vi "Host_GUI.vi"() -> ()   [LabVIEW 2017]
uses:
  <vilib>/Utility/miscctls.llb/LV3DPointTypeDef.ctl
  <vilib>/Analysis/coordinate.llb/Euler Rotation Order.ctl
  <vilib>/picture/3D Picture Control/Object/Create Object (drawable).vi
  <vilib>/picture/3D Picture Control/Object/Create Object (name).vi
  <vilib>/picture/3D Picture Control/Object/Add Object (no reference).vi
  <vilib>/picture/3D Picture Control/Helpers/Apply Texture (no reference).vi
  <vilib>/Analysis/NI_AALPro.lvlib
  <vilib>/picture/3D Picture Control/NI_3D Picture Control.lvlib
  <vilib>/picture/3D Picture Control/Helpers/Set Clip Plane (no reference).vi
panel:
  in  "Up Direction":T1={"X"=0.0, "Y"=0.0, "Z"=1.0}
  out "appended path":path
  in  "error in (no error)":errorcluster
  in  "N-frame rot":dbl[](array[numeric])
  in  "B-frame Translation 2":cluster{"X":sgl, "Y":sgl, "Z":sgl}
  out "B-frame [m]":cluster{"X":sgl, "Y":sgl, "Z":sgl}
  out "Enum":T2(ring)
  in  "Tab Control":enum32{"Inicialização", "Simulação"}(tab)
  in  "Simulation Parameters":T3={"Wind VelocityAzimuth [deg] "=0.0, "Wind Velocity Module [m/s]"=0.0, "Fe gain"=1.0, "Cnalpha gain"=1.0, "clp gain"=1.0, "cld gain"=1.0, "cmq gain"=1.0, "cnr gain"=1.0, "dl [º]"=0.0, "Nozzle misalignment yaw/pitch [º]"=[0.0, 0.0], "Nozzle eccentricity x/y [m]"=[], "Wind_Profile"=0} {"Wind_Profile" min=0 max=3 step=1; "Wind Velocity Module [m/s]" format="%#_13g"; "Wind VelocityAzimuth [deg]" format="%#_13g"}
  in  "Continuar":bool
  in  "stop":bool
  in  "Initialization Parameters":T4={"W_b ini [rad/s]"=[], "W ini [rad/s]"=[], "altitude_ini(m)"=50.0, "lon_ini [º]"=-44.3678, "latd_ini [º]"=-2.31599, "V_ini [m/s]"=[], "Initial Euler Angles [deg]"=[], "CFN-61G Enable"=FALSE, "Table enable"=FALSE, "DMARS Enable"=FALSE, "TVA Enable"=FALSE, "Sim_Time [s]"=82.0, "Control Selection"=enum."Sim Control"}
  out "Euler Angles [deg]":T5(graph)
  in  "Run_SIM":bool
  out "Sim_Stopped":bool
  in  "stop RT":bool
  out "Simulation time [s]":dbl
  out "Atitude":refnum<vi>(3d-picture)
  in  "stop GUI":bool
  out "floor(x/y)":dbl
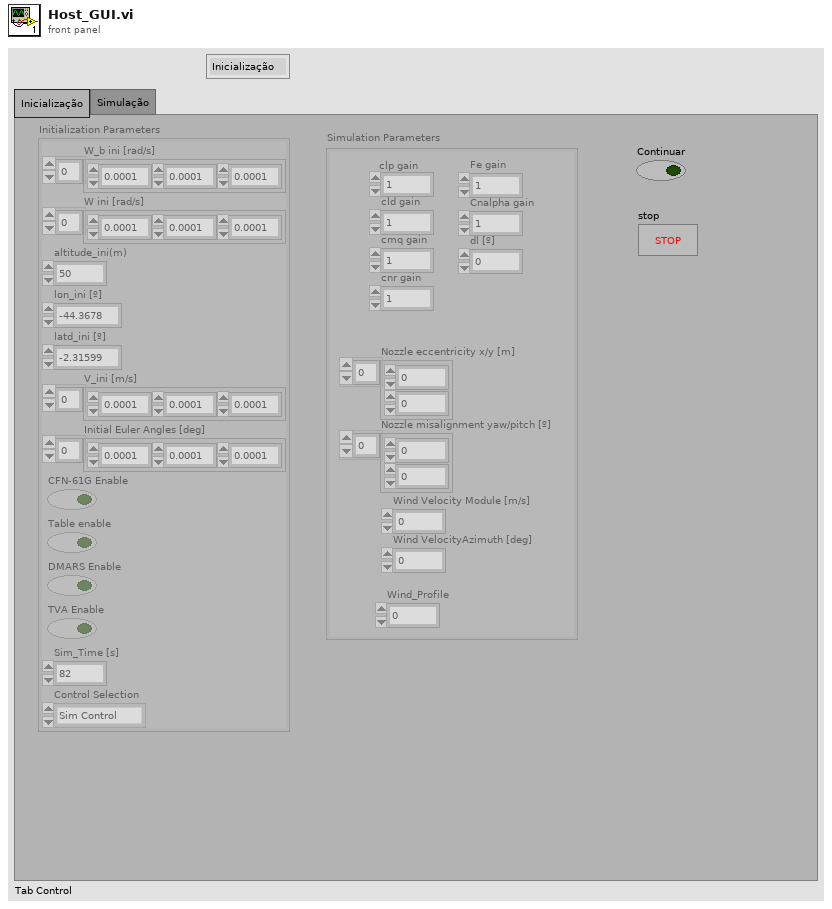
[diagram p1: front panel]
types:
  T1 = typedef "LV3DPointTypeDef.ctl" = cluster{"X":sgl, "Y":sgl, "Z":sgl}
  T2 = enum16{"Inicialização", "Simulação", "Resultados", "Finalizar RT"}
  T3 = cluster{"Wind VelocityAzimuth [deg] ":dbl, "Wind Velocity Module [m/s]":dbl, "Fe gain":dbl, "Cnalpha gain":dbl, "clp gain":dbl, "cld gain":dbl, "cmq gain":dbl, "cnr gain":dbl, "dl [º]":dbl, "Nozzle misalignment yaw/pitch [º]":dbl[], "Nozzle eccentricity x/y [m]":dbl[], "Wind_Profile":i32}
  T4 = cluster{"W_b ini [rad/s]":dbl[], "W ini [rad/s]":dbl[], "altitude_ini(m)":dbl, "lon_ini [º]":dbl, "latd_ini [º]":dbl, "V_ini [m/s]":dbl[], "Initial Euler Angles [deg]":dbl[], "CFN-61G Enable":bool, "Table enable":bool, "DMARS Enable":bool, "TVA Enable":bool, "Sim_Time [s]":dbl, "Control Selection":enum16{"Constant", "TVA E-BOX", "Sim Control"}}
  T5 = cluster{"Numeric":dbl, "Numeric":dbl, "Numeric":dbl}
  T6 = enum16{"As a Decal", "With Modulation", "With Blending", "As a replacement"}
  T7 = cluster{"Red":sgl, "Green":sgl, "Blue":sgl, "Alpha":sgl}
  T8 = enum8{"Enabled", "Disabled", "Disabled and Grayed Out"}
  T9 = typedef "NI_AALPro.lvlib/Euler Rotation Order.ctl" = u16
  T10 = typedef "imagedata.ctl" = cluster{"image type":i32, "image depth":i32, "image":u8[], "mask":u8[], "colors":u32[], "Rectangle":cluster{"left":i16, "top":i16, "right":i16, "bottom":i16}}
  T11 = cluster{"element":dbl, "element":dbl, "element":dbl}
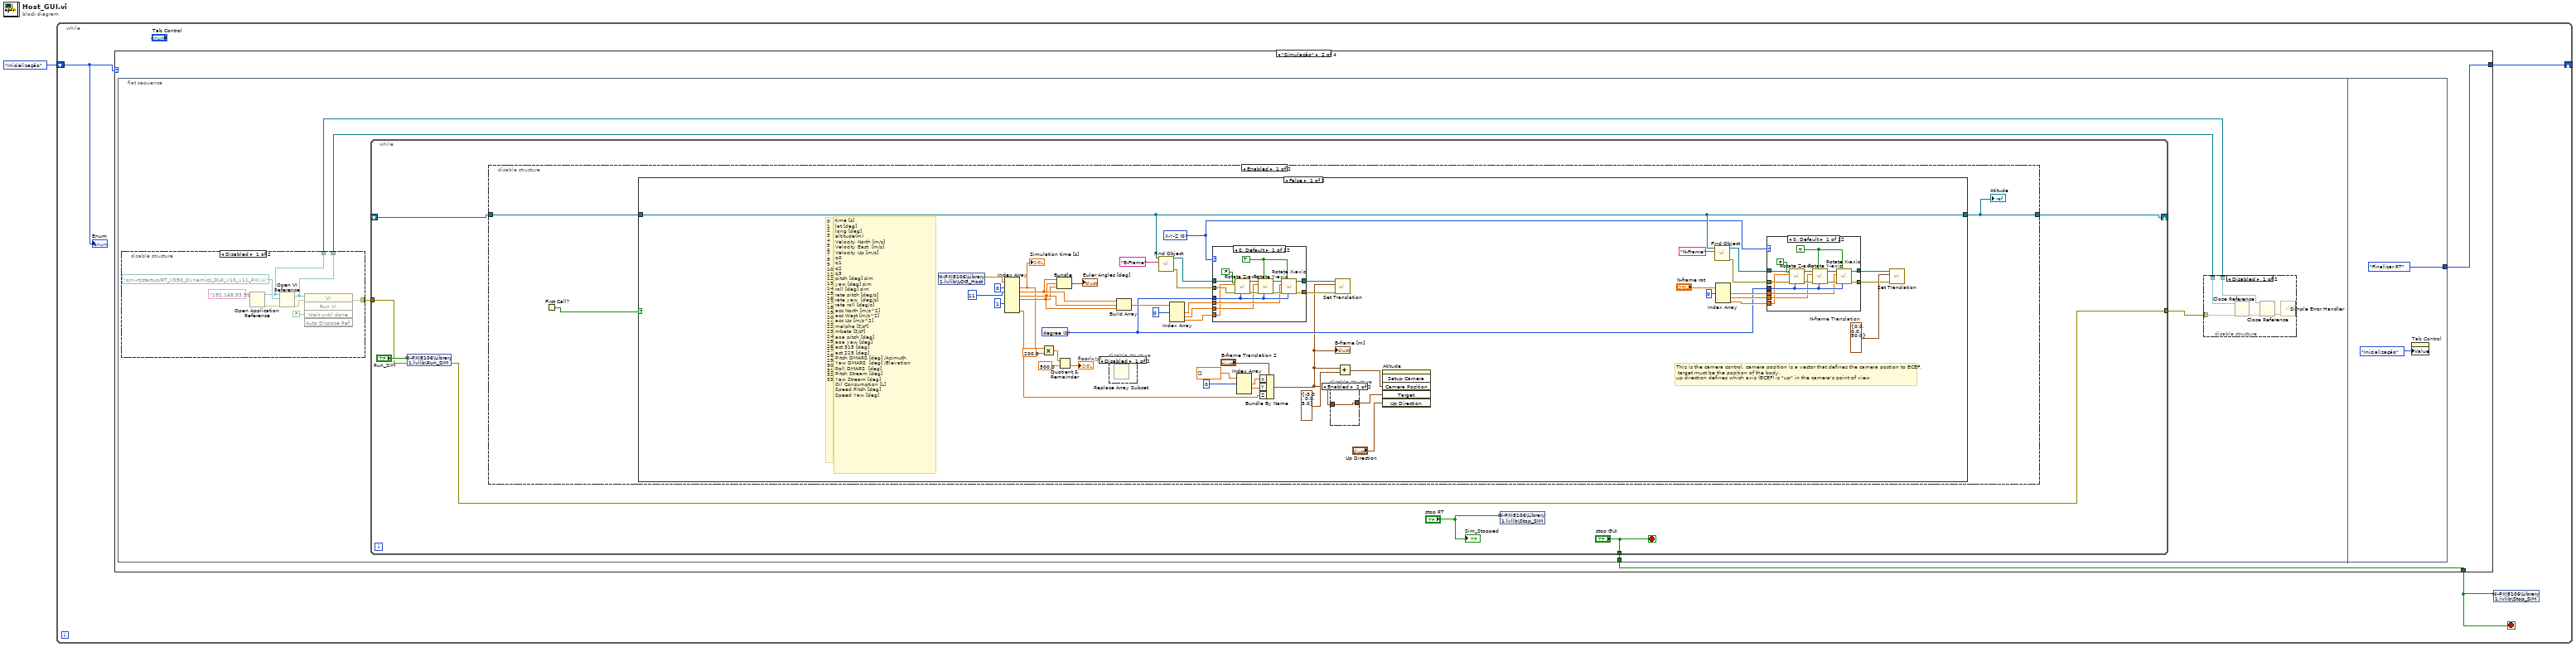
[diagram p0: block diagram]
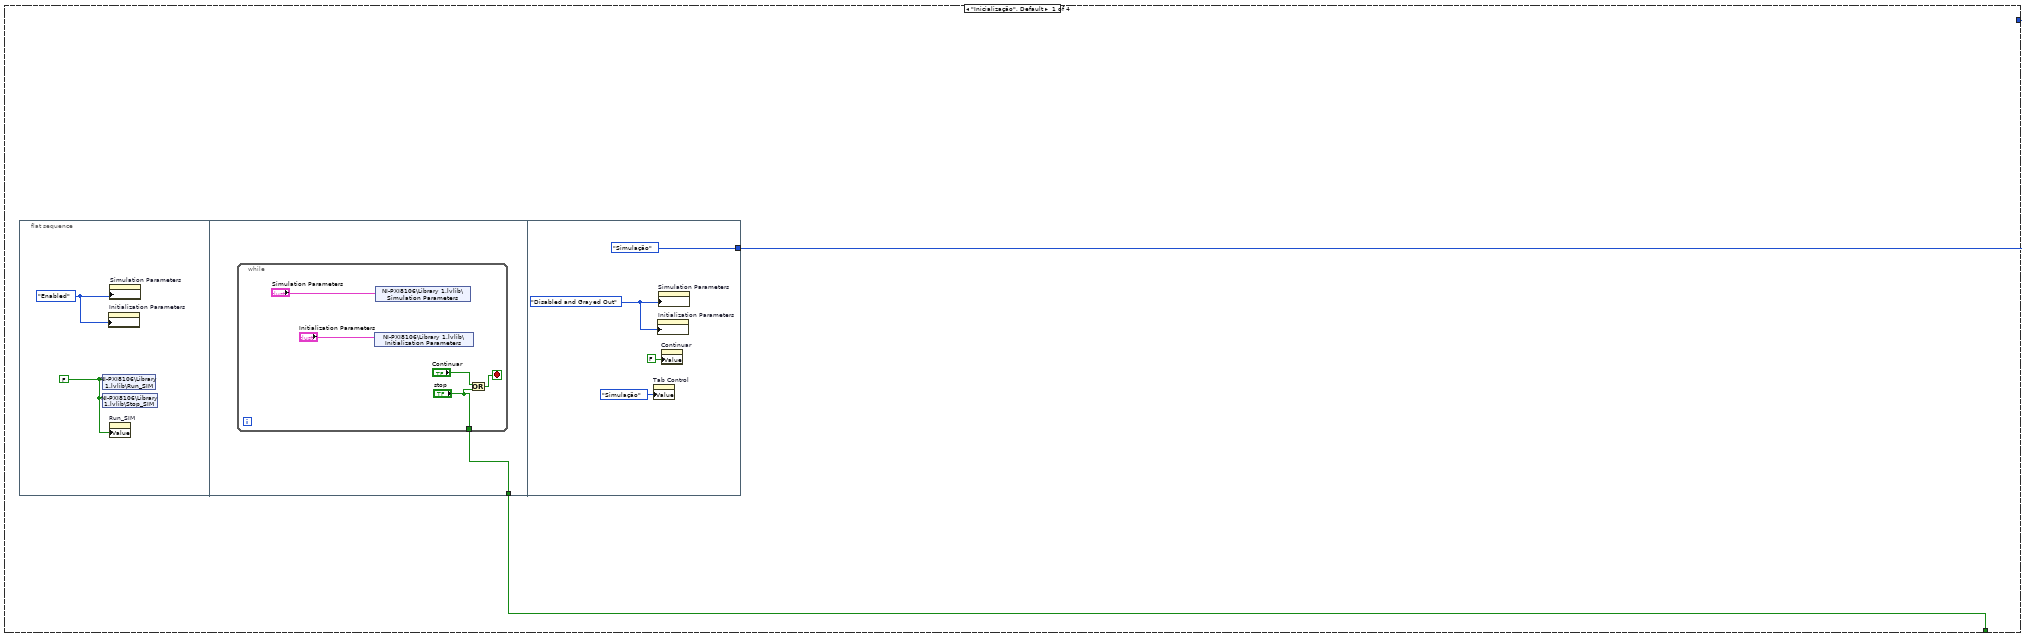
[diagram p2: hidden frame]
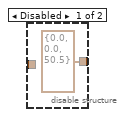
[diagram p6: hidden frame]
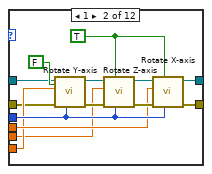
[diagram p7: hidden frame]
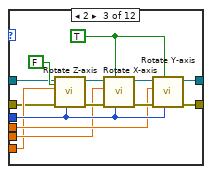
[diagram p8: hidden frame]
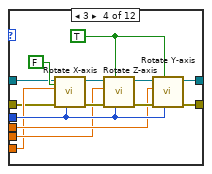
[diagram p9: hidden frame]
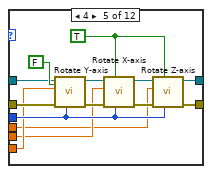
[diagram p10: hidden frame]
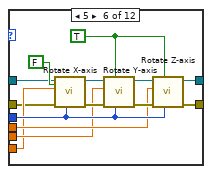
[diagram p11: hidden frame]
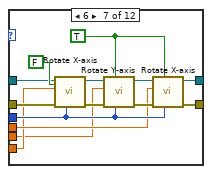
[diagram p12: hidden frame]
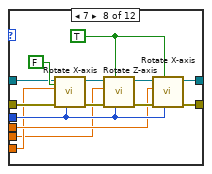
[diagram p13: hidden frame]
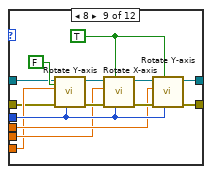
[diagram p14: hidden frame]
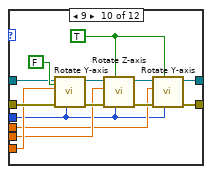
[diagram p15: hidden frame]
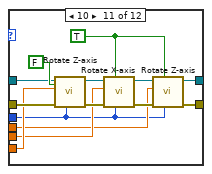
[diagram p16: hidden frame]
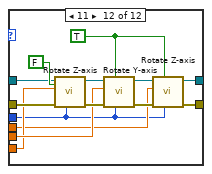
[diagram p17: hidden frame]
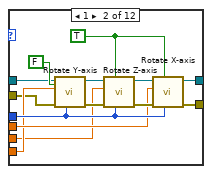
[diagram p18: hidden frame]
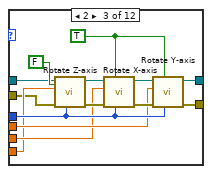
[diagram p19: hidden frame]
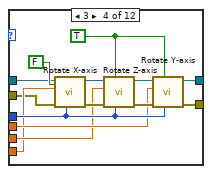
[diagram p20: hidden frame]
diagram:
  n1 = while {
    shift-right: [w4] -> _
    shift-left: T2."Inicialização" -> [w3]
    stop <- w2 stop-if-true
    n2 = case shown="\"Simulação\"" w3 {
      tunnel: [w6 w20 _ _] -> w4
      tunnel: [w5 w19 TRUE ("stop GUI") TRUE ("stop GUI")] -> w2
      frame "Inicialização", Default {
        n3 = flat-sequence {
          tunnel: [w9] -> w5
          tunnel: [T2."Simulação"] -> w6
          frame #0 {
            w8 = FALSE ("Run_SIM")
            w7 = T8."Enabled" ("Disabled")
            n4 = shared-variable "NI-PXI8106\\Library 1.lvlib\\Run_SIM"(w8) -> ()  [unwired: 1 in, 1 out]
            n5 = shared-variable "NI-PXI8106\\Library 1.lvlib\\Stop_SIM"(w8) -> ()  [unwired: 1 in, 1 out]
            n6 = property on="Initialization Parameters" class="Clust (strict)"("DisabledEnum"=w7) -> ()  [unwired: 2 in, 2 out]
            n7 = property on="Run_SIM" class="Bool (strict)"("Value"=w8) -> ()  [unwired: 2 in, 2 out]
            n8 = property on="Simulation Parameters" class="Clust (strict)"("DisabledEnum"=w7) -> ()  [unwired: 2 in, 2 out]
          }
          frame #1 {
            n9 = while {
              tunnel: ["stop"] -> w9
              stop <- w11 stop-if-true
              n10 = shared-variable "NI-PXI8106\\Library 1.lvlib\\Initialization Parameters"("Initialization Parameters") -> ()  [unwired: 1 in, 1 out]
              n11 = shared-variable "NI-PXI8106\\Library 1.lvlib\\Simulation Parameters"("Simulation Parameters") -> ()  [unwired: 1 in, 1 out]
              n12 = Or(x="Continuar", y="stop") -> (x .or. y?=w11:bool)
            }
          }
          frame #2 {
            w15 = T8."Disabled and Grayed Out" ("Disabled")
            n13 = property on="Tab Control" class="TabCtl (strict)"("Value"=enum32{"Inicialização", "Simulação"}."Simulação" ("Tab Control")) -> ()  [unwired: 2 in, 2 out]
            n14 = property on="Initialization Parameters" class="Clust (strict)"("DisabledEnum"=w15) -> ()  [unwired: 2 in, 2 out]
            n15 = property on="Simulation Parameters" class="Clust (strict)"("DisabledEnum"=w15) -> ()  [unwired: 2 in, 2 out]
            n16 = property on="Continuar" class="Bool (strict)"("Value"=FALSE ("Continuar")) -> ()  [unwired: 2 in, 2 out]
          }
        }
      }
      frame "Simulação" {
        n17 = flat-sequence {
          tunnel: [w21] -> w19
          tunnel: [T2."Finalizar RT"] -> w20
          frame #0 {
            n18 = disable-structure shown="Disabled" {
              disable-tunnel: [w33 _] -> w25
              disable-tunnel: [w32 _] -> w24
              disable-tunnel: [w31 _] -> w23
              frame Disabled {
                n19 = Open Application Reference(11:"192.168.53.51" ("machine name (\"\":  open local reference)")) -> (0:w36:errorcluster, 3:w31:refnum<vi>)  [unwired: 3 in]
                n20 = Open VI Reference(application reference (local)=w31, vi path=path "c:/ni-rt/startup/RT_VS50_Dynamics_DLR_v10_v11_PXI.vi", error in (no error)=w36) -> (vi reference=w32:refnum<vi>, error out=w35:errorcluster)  [unwired: 3 in]
                n21 = invoke class="VI" method="Run VI"(reference=w32, error in=w35, "Wait until done"=FALSE ("Wait Until Done")) -> (error out=w33:errorcluster)  [unwired: 2 in, 4 out]
              }
              frame Enabled {
              }
            }
            n22 = while {
              tunnel: w25 -> [w44]
              tunnel: [w43] -> w22
              tunnel: ["stop GUI"] -> w21
              shift-right: [w41] -> _
              shift-left: _ -> [w42]
              stop <- "stop GUI" stop-if-true
              n23 = shared-variable "NI-PXI8106\\Library 1.lvlib\\Run_SIM"("Run_SIM", error in=w44) -> (error out=w43:errorcluster)
              n24 = disable-structure shown="Enabled" {
                disable-tunnel: w42 -> [w48 _]
                disable-tunnel: [w47 _] -> w41
                frame Enabled {
                  n25 = First Call?() -> (First Call?: T/F=w46:bool)
                  n26 = case shown="False" w46 {
                    tunnel: [w77 w450] -> w47
                    tunnel: w48 -> [w77 _]
                    frame False {
                      w76 = T9 0 items=["X-Y-Z", "X-Z-Y", "Y-X-Z", "Y-Z-X", "Z-X-Y", "Z-Y-X", "X-Y-X", "X-Z-X", "Y-X-Y", "Y-Z-Y", "Z-X-Z", "Z-Y-Z"] ("rotation order")
                      w87 = cluster{"X":sgl, "Y":sgl, "Z":sgl} {"X"=0.0, "Y"=0.0, "Z"=50.0}  # N-frame Translation
                      w75 = u16 0 items=["degree", "radians"] ("angle unit")
                      # "0\n1\n2\n3\n4\n5\n6\n7\n8\n9\n10\n11\n12\n13\n14\n15\n16\n17\n18\n19\n20\n21\n22\n23\n24\n25\n26\n27\n28\n29\n30\n31\n32\n33"
                      # "time [s]\nlat [deg]\nlong [deg]\naltitude(m)\nVelocity North [m/s]\nVelocity East  [m/s]\nVelocity Up [m/s]\nq0\nq1\nq2\nq3\npitch [deg] sim\nyaw [deg] sim\nroll [deg] sim\nrate pitch [deg/s] \nrate yaw  [deg/s]\nrate roll [deg/s]\nacc North [m/s^2] \nacc West [m/s^2]\nacc Up [m/s^2]\nmalpha [º/s²]\nmbeta [º/s²]\naoa pitch [deg] \naoa yaw [deg]\nact 315 [deg] \nact 225 [deg]\nPitch DMARS [deg] /Azimuth\nYaw DMARS  [deg] /Elevation\nRoll DMARS  [deg]\nPitch Stream [deg]\nYaw Stream [deg]\nOil Consumption [L]\nSpeed Pitch [deg]\nSpeed Yaw [deg]"
                      # "This is the camera control, camera position is a vector that defines the camera postion to ECEF,\n target must be the position of the body. \nup direction defines which axis (ECEF) is \"up\" in the camera's point of view"
                      n27 = shared-variable "NI-PXI8106\\Library 1.lvlib\\LOG_Host"() -> (w65:dbl[])  [unwired: 1 in, 1 out]
                      n28 = Index Array(array=w65, index #1=0 ("index"), index #2=11 ("index"), index #5=1 ("index")) -> (element #1=w52:dbl, element #2=w57:dbl, element #3=w56:dbl, element #4=w55:dbl, element #7=w59:dbl)  [unwired: 4 in, 2 out]
                      "Simulation time [s]" <- w52
                      n29 = Multiply(x=w52, y=200.0) -> (x*y=w50:dbl)
                      n30 = Bundle("Numeric"=w57, "Numeric"=w56, "Numeric"=w55) -> (→"Euler Angles [deg]":T5)  [unwired: 1 in]
                      n31 = Quotient & Remainder(x=w50, y=500.0) -> (floor(x/y)=→"floor(x/y)":dbl)  [unwired: 1 out]
                      n32 = disable-structure shown="Disabled" {
                        frame Disabled {
                          n33 = Replace Array Subset() -> ()  [unwired: 3 in, 1 out]
                        }
                        frame Enabled {
                        }
                      }
                      n34 = Build Array(w57, w56, w55) -> (w58:dbl[])
                      n35 = call <vilib>:"Find Object.vi"("Object Name"="B-Frame", "Scene Refnum"=w77) -> ("error out"=w93:errorcluster, "Object Refnum"=w94:refnum<vi>)  [unwired: 8 in]
                      n36 = Index Array(array=w58, index #1=0 ("index")) -> (element #1=w95:dbl, element #2=w92:dbl, element #3=w91:dbl)  [unwired: 2 in]
                      n37 = case shown="0, Default" w76 {
                        tunnel: w95 -> [w271 w287 w301 w315 w325 w343 w357 w371 w385 w396 w410 w424]
                        tunnel: w94 -> [w274 w284 w297 w311 w329 w339 w356 w370 w381 w400 w414 w428]
                        tunnel: w93 -> [w273 w283 w298 w312 w328 w340 w355 w369 w382 w399 w413 w427]
                        tunnel: w92 -> [w270 w285 w300 w314 w326 w342 w353 w367 w384 w397 w411 w426]
                        tunnel: w91 -> [w269 w286 w299 w313 w327 w341 w354 w368 w383 w398 w412 w425]
                        tunnel: w75 -> [w272 w288 w302 w316 w330 w344 w358 w372 w386 w395 w409 w423]
                        tunnel: [w268 w282 w296 w310 w324 w338 w352 w366 w380 w394 w408 w422] -> w89
                        tunnel: [w267 w281 w295 w309 w323 w337 w351 w365 w379 w393 w407 w421] -> w88
                        frame 0, Default {
                          w280 = TRUE ("Relative?")
                          n38 = call <vilib>:"Rotate Z-axis.vi"("angle unit"=w272, "Relative?"=FALSE, "error in (no error)"=w273, "angle"=w269, "Scene Object In"=w274) -> ("error out"=w277:errorcluster, "Scene Object Out"=w278:refnum<vi>)  [unwired: 5 in]
                          n39 = call <vilib>:"Rotate Y-axis.vi"("angle unit"=w272, "Relative?"=w280, "error in (no error)"=w277, "angle"=w270, "Scene Object In"=w278) -> ("error out"=w276:errorcluster, "Scene Object Out"=w275:refnum<vi>)  [unwired: 5 in]
                          n40 = call <vilib>:"Rotate X-axis.vi"("angle unit"=w272, "Relative?"=w280, "error in (no error)"=w276, "angle"=w271, "Scene Object In"=w275) -> ("error out"=w267:errorcluster, "Scene Object Out"=w268:refnum<vi>)  [unwired: 5 in]
                        }
                        frame 1 {
                          w291 = TRUE ("Relative?")
                          n41 = call <vilib>:"Rotate Y-axis.vi"("angle unit"=w288, "Relative?"=FALSE, "error in (no error)"=w283, "angle"=w286, "Scene Object In"=w284) -> ("error out"=w292:errorcluster, "Scene Object Out"=w293:refnum<vi>)  [unwired: 5 in]
                          n42 = call <vilib>:"Rotate Z-axis.vi"("angle unit"=w288, "Relative?"=w291, "error in (no error)"=w292, "angle"=w285, "Scene Object In"=w293) -> ("error out"=w289:errorcluster, "Scene Object Out"=w290:refnum<vi>)  [unwired: 5 in]
                          n43 = call <vilib>:"Rotate X-axis.vi"("angle unit"=w288, "Relative?"=w291, "error in (no error)"=w289, "angle"=w287, "Scene Object In"=w290) -> ("error out"=w281:errorcluster, "Scene Object Out"=w282:refnum<vi>)  [unwired: 5 in]
                        }
                        frame 2 {
                          w303 = TRUE ("Relative?")
                          n44 = call <vilib>:"Rotate Z-axis.vi"("angle unit"=w302, "Relative?"=FALSE, "error in (no error)"=w298, "angle"=w299, "Scene Object In"=w297) -> ("error out"=w306:errorcluster, "Scene Object Out"=w307:refnum<vi>)  [unwired: 5 in]
                          n45 = call <vilib>:"Rotate X-axis.vi"("angle unit"=w302, "Relative?"=w303, "error in (no error)"=w306, "angle"=w300, "Scene Object In"=w307) -> ("error out"=w304:errorcluster, "Scene Object Out"=w305:refnum<vi>)  [unwired: 5 in]
                          n46 = call <vilib>:"Rotate Y-axis.vi"("angle unit"=w302, "Relative?"=w303, "error in (no error)"=w304, "angle"=w301, "Scene Object In"=w305) -> ("error out"=w295:errorcluster, "Scene Object Out"=w296:refnum<vi>)  [unwired: 5 in]
                        }
                        frame 3 {
                          w321 = TRUE ("Relative?")
                          n47 = call <vilib>:"Rotate X-axis.vi"("angle unit"=w316, "Relative?"=FALSE, "error in (no error)"=w312, "angle"=w313, "Scene Object In"=w311) -> ("error out"=w319:errorcluster, "Scene Object Out"=w320:refnum<vi>)  [unwired: 5 in]
                          n48 = call <vilib>:"Rotate Z-axis.vi"("angle unit"=w316, "Relative?"=w321, "error in (no error)"=w319, "angle"=w314, "Scene Object In"=w320) -> ("error out"=w317:errorcluster, "Scene Object Out"=w318:refnum<vi>)  [unwired: 5 in]
                          n49 = call <vilib>:"Rotate Y-axis.vi"("angle unit"=w316, "Relative?"=w321, "error in (no error)"=w317, "angle"=w315, "Scene Object In"=w318) -> ("error out"=w309:errorcluster, "Scene Object Out"=w310:refnum<vi>)  [unwired: 5 in]
                        }
                        frame 4 {
                          w335 = TRUE ("Relative?")
                          n50 = call <vilib>:"Rotate Y-axis.vi"("angle unit"=w330, "Relative?"=FALSE, "error in (no error)"=w328, "angle"=w327, "Scene Object In"=w329) -> ("error out"=w331:errorcluster, "Scene Object Out"=w332:refnum<vi>)  [unwired: 5 in]
                          n51 = call <vilib>:"Rotate X-axis.vi"("angle unit"=w330, "Relative?"=w335, "error in (no error)"=w331, "angle"=w326, "Scene Object In"=w332) -> ("error out"=w334:errorcluster, "Scene Object Out"=w333:refnum<vi>)  [unwired: 5 in]
                          n52 = call <vilib>:"Rotate Z-axis.vi"("angle unit"=w330, "Relative?"=w335, "error in (no error)"=w334, "angle"=w325, "Scene Object In"=w333) -> ("error out"=w323:errorcluster, "Scene Object Out"=w324:refnum<vi>)  [unwired: 5 in]
                        }
                        frame 5 {
                          w348 = TRUE ("Relative?")
                          n53 = call <vilib>:"Rotate X-axis.vi"("angle unit"=w344, "Relative?"=FALSE, "error in (no error)"=w340, "angle"=w341, "Scene Object In"=w339) -> ("error out"=w346:errorcluster, "Scene Object Out"=w347:refnum<vi>)  [unwired: 5 in]
                          n54 = call <vilib>:"Rotate Y-axis.vi"("angle unit"=w344, "Relative?"=w348, "error in (no error)"=w346, "angle"=w342, "Scene Object In"=w347) -> ("error out"=w350:errorcluster, "Scene Object Out"=w349:refnum<vi>)  [unwired: 5 in]
                          n55 = call <vilib>:"Rotate Z-axis.vi"("angle unit"=w344, "Relative?"=w348, "error in (no error)"=w350, "angle"=w343, "Scene Object In"=w349) -> ("error out"=w337:errorcluster, "Scene Object Out"=w338:refnum<vi>)  [unwired: 5 in]
                        }
                        frame 6 {
                          w361 = TRUE ("Relative?")
                          n56 = call <vilib>:"Rotate X-axis.vi"("angle unit"=w358, "Relative?"=FALSE, "error in (no error)"=w355, "angle"=w354, "Scene Object In"=w356) -> ("error out"=w363:errorcluster, "Scene Object Out"=w364:refnum<vi>)  [unwired: 5 in]
                          n57 = call <vilib>:"Rotate Y-axis.vi"("angle unit"=w358, "Relative?"=w361, "error in (no error)"=w363, "angle"=w353, "Scene Object In"=w364) -> ("error out"=w359:errorcluster, "Scene Object Out"=w360:refnum<vi>)  [unwired: 5 in]
                          n58 = call <vilib>:"Rotate X-axis.vi"("angle unit"=w358, "Relative?"=w361, "error in (no error)"=w359, "angle"=w357, "Scene Object In"=w360) -> ("error out"=w351:errorcluster, "Scene Object Out"=w352:refnum<vi>)  [unwired: 5 in]
                        }
                        frame 7 {
                          w377 = TRUE ("Relative?")
                          n59 = call <vilib>:"Rotate X-axis.vi"("angle unit"=w372, "Relative?"=FALSE, "error in (no error)"=w369, "angle"=w368, "Scene Object In"=w370) -> ("error out"=w375:errorcluster, "Scene Object Out"=w376:refnum<vi>)  [unwired: 5 in]
                          n60 = call <vilib>:"Rotate Z-axis.vi"("angle unit"=w372, "Relative?"=w377, "error in (no error)"=w375, "angle"=w367, "Scene Object In"=w376) -> ("error out"=w374:errorcluster, "Scene Object Out"=w373:refnum<vi>)  [unwired: 5 in]
                          n61 = call <vilib>:"Rotate X-axis.vi"("angle unit"=w372, "Relative?"=w377, "error in (no error)"=w374, "angle"=w371, "Scene Object In"=w373) -> ("error out"=w365:errorcluster, "Scene Object Out"=w366:refnum<vi>)  [unwired: 5 in]
                        }
                        frame 8 {
                          w391 = TRUE ("Relative?")
                          n62 = call <vilib>:"Rotate Y-axis.vi"("angle unit"=w386, "Relative?"=FALSE, "error in (no error)"=w382, "angle"=w383, "Scene Object In"=w381) -> ("error out"=w389:errorcluster, "Scene Object Out"=w390:refnum<vi>)  [unwired: 5 in]
                          n63 = call <vilib>:"Rotate X-axis.vi"("angle unit"=w386, "Relative?"=w391, "error in (no error)"=w389, "angle"=w384, "Scene Object In"=w390) -> ("error out"=w388:errorcluster, "Scene Object Out"=w387:refnum<vi>)  [unwired: 5 in]
                          n64 = call <vilib>:"Rotate Y-axis.vi"("angle unit"=w386, "Relative?"=w391, "error in (no error)"=w388, "angle"=w385, "Scene Object In"=w387) -> ("error out"=w379:errorcluster, "Scene Object Out"=w380:refnum<vi>)  [unwired: 5 in]
                        }
                        frame 9 {
                          w405 = TRUE ("Relative?")
                          n65 = call <vilib>:"Rotate Y-axis.vi"("angle unit"=w395, "Relative?"=FALSE, "error in (no error)"=w399, "angle"=w398, "Scene Object In"=w400) -> ("error out"=w403:errorcluster, "Scene Object Out"=w404:refnum<vi>)  [unwired: 5 in]
                          n66 = call <vilib>:"Rotate Z-axis.vi"("angle unit"=w395, "Relative?"=w405, "error in (no error)"=w403, "angle"=w397, "Scene Object In"=w404) -> ("error out"=w402:errorcluster, "Scene Object Out"=w401:refnum<vi>)  [unwired: 5 in]
                          n67 = call <vilib>:"Rotate Y-axis.vi"("angle unit"=w395, "Relative?"=w405, "error in (no error)"=w402, "angle"=w396, "Scene Object In"=w401) -> ("error out"=w393:errorcluster, "Scene Object Out"=w394:refnum<vi>)  [unwired: 5 in]
                        }
                        frame 10 {
                          w419 = TRUE ("Relative?")
                          n68 = call <vilib>:"Rotate Z-axis.vi"("angle unit"=w409, "Relative?"=FALSE, "error in (no error)"=w413, "angle"=w412, "Scene Object In"=w414) -> ("error out"=w417:errorcluster, "Scene Object Out"=w418:refnum<vi>)  [unwired: 5 in]
                          n69 = call <vilib>:"Rotate X-axis.vi"("angle unit"=w409, "Relative?"=w419, "error in (no error)"=w417, "angle"=w411, "Scene Object In"=w418) -> ("error out"=w416:errorcluster, "Scene Object Out"=w415:refnum<vi>)  [unwired: 5 in]
                          n70 = call <vilib>:"Rotate Z-axis.vi"("angle unit"=w409, "Relative?"=w419, "error in (no error)"=w416, "angle"=w410, "Scene Object In"=w415) -> ("error out"=w407:errorcluster, "Scene Object Out"=w408:refnum<vi>)  [unwired: 5 in]
                        }
                        frame 11 {
                          w433 = TRUE ("Relative?")
                          n71 = call <vilib>:"Rotate Z-axis.vi"("angle unit"=w423, "Relative?"=FALSE, "error in (no error)"=w427, "angle"=w425, "Scene Object In"=w428) -> ("error out"=w431:errorcluster, "Scene Object Out"=w432:refnum<vi>)  [unwired: 5 in]
                          n72 = call <vilib>:"Rotate Y-axis.vi"("angle unit"=w423, "Relative?"=w433, "error in (no error)"=w431, "angle"=w426, "Scene Object In"=w432) -> ("error out"=w430:errorcluster, "Scene Object Out"=w429:refnum<vi>)  [unwired: 5 in]
                          n73 = call <vilib>:"Rotate Z-axis.vi"("angle unit"=w423, "Relative?"=w433, "error in (no error)"=w430, "angle"=w424, "Scene Object In"=w429) -> ("error out"=w421:errorcluster, "Scene Object Out"=w422:refnum<vi>)  [unwired: 5 in]
                        }
                      }
                      n74 = Index Array(array=dbl[] [], index #1=0 ("index")) -> (element #1=w72:dbl, element #2=w71:dbl)  [unwired: 2 in, 1 out]
                      n75 = Bundle By Name(cluster="B-frame Translation 2", "X"=w72, "Y"=w71, "Z"=w59) -> (w61:cluster{"X":sgl, "Y":sgl, "Z":sgl})
                      "B-frame [m]" <- w61
                      n76 = disable-structure shown="Enabled" {
                        disable-tunnel: [T1 {"X"=0.0, "Y"=0.0, "Z"=50.5} ("Target") w98] -> w67
                        disable-tunnel: w61 -> [_ w98]
                        frame Disabled {
                        }
                        frame Enabled {
                        }
                      }
                      n77 = call <vilib>:"Set Translation.vi"("error in (no error)"=w88, "Translation"=w61, "Scene Object"=w89) -> ()  [unwired: 7 in, 2 out]
                      n78 = Add(x=w61, y=T1 {"X"=-3.0, "Y"=0.0, "Z"=5.0} ("Camera Position control")) -> (x+y=w60:T1)
                      n79 = invoke on="Atitude" class="SceneGraphDisp (strict)" method="Setup Camera"("Camera Position"=w60, "Target"=w67, "Up Direction"="Up Direction") -> ()  [unwired: 3 in, 6 out]
                      n80 = call <vilib>:"Find Object.vi"("Object Name"="N-Frame", "Scene Refnum"=w77) -> ("error out"=w81:errorcluster, "Object Refnum"=w80:refnum<vi>)  [unwired: 8 in]
                      n81 = Index Array(array="N-frame rot", index #1=0 ("index")) -> (element #1=w79:dbl, element #2=w82:dbl, element #3=w83:dbl)  [unwired: 2 in]
                      n82 = case shown="0, Default" w76 {
                        tunnel: w79 -> [w103 w119 w133 w147 w157 w175 w189 w203 w217 w228 w242 w256]
                        tunnel: w80 -> [w106 w116 w129 w143 w161 w171 w188 w202 w213 w232 w246 w260]
                        tunnel: w81 -> [w105 w115 w130 w144 w160 w172 w187 w201 w214 w231 w245 w259]
                        tunnel: w82 -> [w102 w117 w132 w146 w158 w174 w185 w199 w216 w229 w243 w258]
                        tunnel: w83 -> [w101 w118 w131 w145 w159 w173 w186 w200 w215 w230 w244 w257]
                        tunnel: w75 -> [w104 w120 w134 w148 w162 w176 w190 w204 w218 w227 w241 w255]
                        tunnel: [w100 w114 w128 w142 w156 w170 w184 w198 w212 w226 w240 w254] -> w85
                        tunnel: [w99 w113 w127 w141 w155 w169 w183 w197 w211 w225 w239 w253] -> w86
                        frame 0, Default {
                          w112 = TRUE ("Relative?")
                          n83 = call <vilib>:"Rotate Z-axis.vi"("angle unit"=w104, "Relative?"=FALSE, "error in (no error)"=w105, "angle"=w101, "Scene Object In"=w106) -> ("error out"=w109:errorcluster, "Scene Object Out"=w110:refnum<vi>)  [unwired: 5 in]
                          n84 = call <vilib>:"Rotate Y-axis.vi"("angle unit"=w104, "Relative?"=w112, "error in (no error)"=w109, "angle"=w102, "Scene Object In"=w110) -> ("error out"=w108:errorcluster, "Scene Object Out"=w107:refnum<vi>)  [unwired: 5 in]
                          n85 = call <vilib>:"Rotate X-axis.vi"("angle unit"=w104, "Relative?"=w112, "error in (no error)"=w108, "angle"=w103, "Scene Object In"=w107) -> ("error out"=w99:errorcluster, "Scene Object Out"=w100:refnum<vi>)  [unwired: 5 in]
                        }
                        frame 1 {
                          w123 = TRUE ("Relative?")
                          n86 = call <vilib>:"Rotate Y-axis.vi"("angle unit"=w120, "Relative?"=FALSE, "error in (no error)"=w115, "angle"=w118, "Scene Object In"=w116) -> ("error out"=w124:errorcluster, "Scene Object Out"=w125:refnum<vi>)  [unwired: 5 in]
                          n87 = call <vilib>:"Rotate Z-axis.vi"("angle unit"=w120, "Relative?"=w123, "error in (no error)"=w124, "angle"=w117, "Scene Object In"=w125) -> ("error out"=w121:errorcluster, "Scene Object Out"=w122:refnum<vi>)  [unwired: 5 in]
                          n88 = call <vilib>:"Rotate X-axis.vi"("angle unit"=w120, "Relative?"=w123, "error in (no error)"=w121, "angle"=w119, "Scene Object In"=w122) -> ("error out"=w113:errorcluster, "Scene Object Out"=w114:refnum<vi>)  [unwired: 5 in]
                        }
                        frame 2 {
                          w135 = TRUE ("Relative?")
                          n89 = call <vilib>:"Rotate Z-axis.vi"("angle unit"=w134, "Relative?"=FALSE, "error in (no error)"=w130, "angle"=w131, "Scene Object In"=w129) -> ("error out"=w138:errorcluster, "Scene Object Out"=w139:refnum<vi>)  [unwired: 5 in]
                          n90 = call <vilib>:"Rotate X-axis.vi"("angle unit"=w134, "Relative?"=w135, "error in (no error)"=w138, "angle"=w132, "Scene Object In"=w139) -> ("error out"=w136:errorcluster, "Scene Object Out"=w137:refnum<vi>)  [unwired: 5 in]
                          n91 = call <vilib>:"Rotate Y-axis.vi"("angle unit"=w134, "Relative?"=w135, "error in (no error)"=w136, "angle"=w133, "Scene Object In"=w137) -> ("error out"=w127:errorcluster, "Scene Object Out"=w128:refnum<vi>)  [unwired: 5 in]
                        }
                        frame 3 {
                          w153 = TRUE ("Relative?")
                          n92 = call <vilib>:"Rotate X-axis.vi"("angle unit"=w148, "Relative?"=FALSE, "error in (no error)"=w144, "angle"=w145, "Scene Object In"=w143) -> ("error out"=w151:errorcluster, "Scene Object Out"=w152:refnum<vi>)  [unwired: 5 in]
                          n93 = call <vilib>:"Rotate Z-axis.vi"("angle unit"=w148, "Relative?"=w153, "error in (no error)"=w151, "angle"=w146, "Scene Object In"=w152) -> ("error out"=w149:errorcluster, "Scene Object Out"=w150:refnum<vi>)  [unwired: 5 in]
                          n94 = call <vilib>:"Rotate Y-axis.vi"("angle unit"=w148, "Relative?"=w153, "error in (no error)"=w149, "angle"=w147, "Scene Object In"=w150) -> ("error out"=w141:errorcluster, "Scene Object Out"=w142:refnum<vi>)  [unwired: 5 in]
                        }
                        frame 4 {
                          w167 = TRUE ("Relative?")
                          n95 = call <vilib>:"Rotate Y-axis.vi"("angle unit"=w162, "Relative?"=FALSE, "error in (no error)"=w160, "angle"=w159, "Scene Object In"=w161) -> ("error out"=w163:errorcluster, "Scene Object Out"=w164:refnum<vi>)  [unwired: 5 in]
                          n96 = call <vilib>:"Rotate X-axis.vi"("angle unit"=w162, "Relative?"=w167, "error in (no error)"=w163, "angle"=w158, "Scene Object In"=w164) -> ("error out"=w166:errorcluster, "Scene Object Out"=w165:refnum<vi>)  [unwired: 5 in]
                          n97 = call <vilib>:"Rotate Z-axis.vi"("angle unit"=w162, "Relative?"=w167, "error in (no error)"=w166, "angle"=w157, "Scene Object In"=w165) -> ("error out"=w155:errorcluster, "Scene Object Out"=w156:refnum<vi>)  [unwired: 5 in]
                        }
                        frame 5 {
                          w180 = TRUE ("Relative?")
                          n98 = call <vilib>:"Rotate X-axis.vi"("angle unit"=w176, "Relative?"=FALSE, "error in (no error)"=w172, "angle"=w173, "Scene Object In"=w171) -> ("error out"=w178:errorcluster, "Scene Object Out"=w179:refnum<vi>)  [unwired: 5 in]
                          n99 = call <vilib>:"Rotate Y-axis.vi"("angle unit"=w176, "Relative?"=w180, "error in (no error)"=w178, "angle"=w174, "Scene Object In"=w179) -> ("error out"=w182:errorcluster, "Scene Object Out"=w181:refnum<vi>)  [unwired: 5 in]
                          n100 = call <vilib>:"Rotate Z-axis.vi"("angle unit"=w176, "Relative?"=w180, "error in (no error)"=w182, "angle"=w175, "Scene Object In"=w181) -> ("error out"=w169:errorcluster, "Scene Object Out"=w170:refnum<vi>)  [unwired: 5 in]
                        }
                        frame 6 {
                          w193 = TRUE ("Relative?")
                          n101 = call <vilib>:"Rotate X-axis.vi"("angle unit"=w190, "Relative?"=FALSE, "error in (no error)"=w187, "angle"=w186, "Scene Object In"=w188) -> ("error out"=w195:errorcluster, "Scene Object Out"=w196:refnum<vi>)  [unwired: 5 in]
                          n102 = call <vilib>:"Rotate Y-axis.vi"("angle unit"=w190, "Relative?"=w193, "error in (no error)"=w195, "angle"=w185, "Scene Object In"=w196) -> ("error out"=w191:errorcluster, "Scene Object Out"=w192:refnum<vi>)  [unwired: 5 in]
                          n103 = call <vilib>:"Rotate X-axis.vi"("angle unit"=w190, "Relative?"=w193, "error in (no error)"=w191, "angle"=w189, "Scene Object In"=w192) -> ("error out"=w183:errorcluster, "Scene Object Out"=w184:refnum<vi>)  [unwired: 5 in]
                        }
                        frame 7 {
                          w209 = TRUE ("Relative?")
                          n104 = call <vilib>:"Rotate X-axis.vi"("angle unit"=w204, "Relative?"=FALSE, "error in (no error)"=w201, "angle"=w200, "Scene Object In"=w202) -> ("error out"=w207:errorcluster, "Scene Object Out"=w208:refnum<vi>)  [unwired: 5 in]
                          n105 = call <vilib>:"Rotate Z-axis.vi"("angle unit"=w204, "Relative?"=w209, "error in (no error)"=w207, "angle"=w199, "Scene Object In"=w208) -> ("error out"=w206:errorcluster, "Scene Object Out"=w205:refnum<vi>)  [unwired: 5 in]
                          n106 = call <vilib>:"Rotate X-axis.vi"("angle unit"=w204, "Relative?"=w209, "error in (no error)"=w206, "angle"=w203, "Scene Object In"=w205) -> ("error out"=w197:errorcluster, "Scene Object Out"=w198:refnum<vi>)  [unwired: 5 in]
                        }
                        frame 8 {
                          w223 = TRUE ("Relative?")
                          n107 = call <vilib>:"Rotate Y-axis.vi"("angle unit"=w218, "Relative?"=FALSE, "error in (no error)"=w214, "angle"=w215, "Scene Object In"=w213) -> ("error out"=w221:errorcluster, "Scene Object Out"=w222:refnum<vi>)  [unwired: 5 in]
                          n108 = call <vilib>:"Rotate X-axis.vi"("angle unit"=w218, "Relative?"=w223, "error in (no error)"=w221, "angle"=w216, "Scene Object In"=w222) -> ("error out"=w220:errorcluster, "Scene Object Out"=w219:refnum<vi>)  [unwired: 5 in]
                          n109 = call <vilib>:"Rotate Y-axis.vi"("angle unit"=w218, "Relative?"=w223, "error in (no error)"=w220, "angle"=w217, "Scene Object In"=w219) -> ("error out"=w211:errorcluster, "Scene Object Out"=w212:refnum<vi>)  [unwired: 5 in]
                        }
                        frame 9 {
                          w237 = TRUE ("Relative?")
                          n110 = call <vilib>:"Rotate Y-axis.vi"("angle unit"=w227, "Relative?"=FALSE, "error in (no error)"=w231, "angle"=w230, "Scene Object In"=w232) -> ("error out"=w235:errorcluster, "Scene Object Out"=w236:refnum<vi>)  [unwired: 5 in]
                          n111 = call <vilib>:"Rotate Z-axis.vi"("angle unit"=w227, "Relative?"=w237, "error in (no error)"=w235, "angle"=w229, "Scene Object In"=w236) -> ("error out"=w234:errorcluster, "Scene Object Out"=w233:refnum<vi>)  [unwired: 5 in]
                          n112 = call <vilib>:"Rotate Y-axis.vi"("angle unit"=w227, "Relative?"=w237, "error in (no error)"=w234, "angle"=w228, "Scene Object In"=w233) -> ("error out"=w225:errorcluster, "Scene Object Out"=w226:refnum<vi>)  [unwired: 5 in]
                        }
                        frame 10 {
                          w251 = TRUE ("Relative?")
                          n113 = call <vilib>:"Rotate Z-axis.vi"("angle unit"=w241, "Relative?"=FALSE, "error in (no error)"=w245, "angle"=w244, "Scene Object In"=w246) -> ("error out"=w249:errorcluster, "Scene Object Out"=w250:refnum<vi>)  [unwired: 5 in]
                          n114 = call <vilib>:"Rotate X-axis.vi"("angle unit"=w241, "Relative?"=w251, "error in (no error)"=w249, "angle"=w243, "Scene Object In"=w250) -> ("error out"=w248:errorcluster, "Scene Object Out"=w247:refnum<vi>)  [unwired: 5 in]
                          n115 = call <vilib>:"Rotate Z-axis.vi"("angle unit"=w241, "Relative?"=w251, "error in (no error)"=w248, "angle"=w242, "Scene Object In"=w247) -> ("error out"=w239:errorcluster, "Scene Object Out"=w240:refnum<vi>)  [unwired: 5 in]
                        }
                        frame 11 {
                          w265 = TRUE ("Relative?")
                          n116 = call <vilib>:"Rotate Z-axis.vi"("angle unit"=w255, "Relative?"=FALSE, "error in (no error)"=w259, "angle"=w257, "Scene Object In"=w260) -> ("error out"=w263:errorcluster, "Scene Object Out"=w264:refnum<vi>)  [unwired: 5 in]
                          n117 = call <vilib>:"Rotate Y-axis.vi"("angle unit"=w255, "Relative?"=w265, "error in (no error)"=w263, "angle"=w258, "Scene Object In"=w264) -> ("error out"=w262:errorcluster, "Scene Object Out"=w261:refnum<vi>)  [unwired: 5 in]
                          n118 = call <vilib>:"Rotate Z-axis.vi"("angle unit"=w255, "Relative?"=w265, "error in (no error)"=w262, "angle"=w256, "Scene Object In"=w261) -> ("error out"=w253:errorcluster, "Scene Object Out"=w254:refnum<vi>)  [unwired: 5 in]
                        }
                      }
                      n119 = call <vilib>:"Set Translation.vi"("error in (no error)"=w86, "Translation"=w87, "Scene Object"=w85) -> ()  [unwired: 7 in, 2 out]
                    }
                    frame True {
                      w444 = -50.0 ("element")
                      w491 = 100 ("dimension size")
                      w493 = sgl 1.0 ("Row Interval")
                      # "Initial P ECEF"
                      # "Branco"
                      # "Cria o frame do corpo"
                      # "Cria o frame de navegação"
                      # "This loads the texture map and\nreadies it to use on the ground."
                      # "Use the random height matrix\nto generate a height grid."
                      n120 = disable-structure shown="Enabled" {
                        disable-tunnel: [w514 _] -> w487
                        disable-tunnel: [w513 _] -> w480
                        frame Enabled {
                          (unwired) path "C:/Users/ASE-LINCS/Desktop/Cesar Moura/Sim_VS50_lv2017/Lv17/World_Map3.png" ("path")
                          n121 = Current VI's Path() -> (path=w511:path)
                          n122 = Strip Path(path=w511) -> (stripped path=w510:path)  [unwired: 1 out]
                          n123 = Build Path(base path=w510, name or relative path="ground.png") -> (appended path=w509:path)
                          "appended path" <- w509
                          n124 = call <vilib>:"Read PNG File.vi"("path to PNG file"=w509) -> ("error out"=w513:errorcluster, "image data"=w514:T10)  [unwired: 8 in, 1 out]
                        }
                        frame Disabled {
                        }
                      }
                      n125 = Initialize Array(0.0 ("element"), w491, w491) -> (w489:dbl[][])
                      n126 = call <vilib>:"Create Height Field.vi"("Column Interval"=w493, "Row Interval"=w493, "Data"=w489) -> ("error out"=w437:errorcluster, "New Height Field Refnum"=w436:refnum<vi>)  [unwired: 1 in, 6 out]
                      n127 = call-poly <vilib>:"Create Object.vi"("error in (no error)"=w437, "Geometry"=w436, "Name"="Base") -> ("error out"=w435:errorcluster, "Scene:New Object"=w438:refnum<vi>)  [unwired: 7 in]
                      n128 = Merge Errors(w435, w480) -> (w445:errorcluster)
                      n129 = call-poly <vilib>:"Apply Texture.vi"("Horizontal Wrap Mode"=enum16{"Clamp", "Repeat"}."Repeat", "error in (no error)"=w445, "Apply Mode"=T6."As a Decal", "Image Data"=w487, "Scene Object In"=w438) -> ("error out"=w481:errorcluster, "Scene Object Out"=w488:refnum<vi>)  [unwired: 5 in]
                      n130 = Bundle("element"=w444, "element"=w444, "element"=50.0) -> (w492:T11)  [unwired: 1 out]
                      n131 = call <vilib>:"Set Translation.vi"("error in (no error)"=w481, "Translation"=w492, "Scene Object"=w488) -> ("error out"=w482:errorcluster, "Translated Object"=w485:refnum<vi>)  [unwired: 7 out]
                      n132 = call-poly <vilib>:"Create Object.vi"("error in (no error)"="error in (no error)", "Name"="world") -> ("error out"=w483:errorcluster, "Scene:New Object"=w484:refnum<vi>)  [unwired: 8 in]
                      n133 = Merge Errors(w483, w482) -> (w442:errorcluster)
                      n134 = call-poly <vilib>:"Add Object.vi"("error in (no error)"=w442, "New Object In"=w485, "Scene Object In"=w484) -> ("error out"=w440:errorcluster, "Scene Object Out"=w441:refnum<vi>)  [unwired: 7 in]
                      n135 = disable-structure shown="Enabled" {
                        disable-tunnel: [w506 w507] -> w463
                        disable-tunnel: [w505 w508] -> w462
                        disable-tunnel: w441 -> [w495 w508]
                        disable-tunnel: w440 -> [w494 w507]
                        frame Disabled {
                          w504 = sgl 0.0 ("A")
                          # "Underneath Clipping\nPlane: z = 0"
                          n136 = Bundle By Name(cluster=cluster{"A":sgl, "B":sgl, "C":sgl, "D":sgl} {"A"=0.0, "B"=0.0, "C"=0.0, "D"=0.0} ("Plane"), "A"=w504, "B"=w504, "C"=sgl 1.0 ("B"), "D"=sgl 0.01 ("B")) -> (w501:cluster{"A":sgl, "B":sgl, "C":sgl, "D":sgl})
                          n137 = call <vilib>:"Create Clip Plane.vi"("error in (no error)"=w494, "Number"=0, "Plane"=w501) -> ("error out"=w497:errorcluster, "New Clip Plane Refnum"=w499:refnum<vi>)  [unwired: 7 out]
                          n138 = call-poly <vilib>:"Set Clip Plane.vi"("error in (no error)"=w497, "Clip Plane State"=enum16{"Inherit Value", "Off", "On"}."Off", "Clip Plane Refnum In"=w499, "Scene Object In"=w495) -> ("error out"=w506:errorcluster, "Scene Object Out"=w505:refnum<vi>)  [unwired: 6 in]
                        }
                        frame Enabled {
                        }
                      }
                      n139 = call <vilib>:"Create 3D Axis.vi"("Axis label?"=TRUE, "Color"=T7 {"Red"=0.0, "Green"=1.0, "Blue"=0.0, "Alpha"=1.0}, "Length"=sgl 1.0 ("Radius"), "Name"="B-Frame") -> ("error out"=w464:errorcluster, "New Object Refnum"=w465:refnum<vi>)  [unwired: 6 in]
                      n140 = call-poly <vilib>:"Create Object.vi"("Name"="Corpo") -> ("error out"=w458:errorcluster, "Scene:New Object"=w459:refnum<vi>)  [unwired: 9 in]
                      n141 = call <vilib>:"Create 3D Axis.vi"("Axis label?"=TRUE, "Color"=T7 {"Red"=1.0, "Green"=1.0, "Blue"=1.0, "Alpha"=1.0}, "Length"=sgl 1.0 ("Radius"), "Name"="N-Frame") -> ("error out"=w455:errorcluster, "New Object Refnum"=w454:refnum<vi>)  [unwired: 6 in]
                      n142 = call <vilib>:"Set Translation.vi"("error in (no error)"=w458, "Translation"=cluster{"X":sgl, "Y":sgl, "Z":sgl} {"X"=0.0, "Y"=0.0, "Z"=0.0}, "Scene Object"=w459) -> ("error out"=w461:errorcluster, "Translated Object"=w460:refnum<vi>)  [unwired: 7 out]
                      n143 = Merge Errors(w461, w464) -> (w468:errorcluster)
                      n144 = call-poly <vilib>:"Add Object.vi"("error in (no error)"=w468, "New Object In"=w465, "Scene Object In"=w460) -> ("error out"=w466:errorcluster, "Scene Object Out"=w467:refnum<vi>)  [unwired: 7 in]
                      n145 = call <vilib>:"Set Translation.vi"("error in (no error)"=w455, "Translation"=cluster{"X":sgl, "Y":sgl, "Z":sgl} {"X"=0.0, "Y"=0.0, "Z"=0.0}, "Scene Object"=w454) -> ("error out"=w453:errorcluster, "Translated Object"=w452:refnum<vi>)  [unwired: 7 out]
                      n146 = Merge Errors(w463, w466) -> (w478:errorcluster)
                      n147 = call-poly <vilib>:"Add Object.vi"("error in (no error)"=w478, "New Object In"=w467, "Scene Object In"=w462) -> ("error out"=w472:errorcluster, "Scene Object Out"=w475:refnum<vi>)  [unwired: 7 in]
                      n148 = Merge Errors(w472, w453) -> (w471:errorcluster)
                      n149 = call-poly <vilib>:"Add Object.vi"("error in (no error)"=w471, "New Object In"=w452, "Scene Object In"=w475) -> ("Scene Object Out"=w450:refnum<vi>)  [unwired: 7 in, 1 out]
                    }
                  }
                  "Atitude" <- w47
                }
                frame Disabled {
                }
              }
              n150 = shared-variable "NI-PXI8106\\Library 1.lvlib\\Stop_SIM"("stop RT") -> ()  [unwired: 1 in, 1 out]
              "Sim_Stopped" <- "stop RT"
            }
            n151 = disable-structure shown="Disabled" {
              disable-tunnel: w24 -> [w30 _]
              disable-tunnel: w23 -> [w29 _]
              disable-tunnel: w22 -> [w26 _]
              frame Disabled {
                n152 = Close Reference(reference=w30, error in (no error)=w26) -> (error out=w28:errorcluster)
                n153 = Close Reference(reference=w29, error in (no error)=w28) -> (error out=w27:errorcluster)
                n154 = call <vilib>:"Simple Error Handler.vi"("error in (no error)"=w27) -> ()  [unwired: 4 in, 5 out]
              }
              frame Enabled {
              }
            }
          }
          frame #1 {
            n155 = property on="Tab Control" class="TabCtl (strict)"("Value"=enum32{"Inicialização", "Simulação"}."Inicialização" ("Tab Control")) -> ()  [unwired: 2 in, 2 out]
          }
        }
      }
      frame "Resultados" {
      }
      frame "Finalizar RT" {
      }
    }
    n156 = shared-variable "NI-PXI8106\\Library 1.lvlib\\Stop_SIM"(w2) -> ()  [unwired: 1 in, 1 out]
    "Enum" <- w3
  }
